vi "fpga_ARC Filter Info.vi"(1 "resample position [U64.16]":fxp<+,64,16>, 2 "stepsize [U64.8]":fxp<+,64,8>, 4 "input valid":bool, 6 "ARC Constants":T1={"bufsize"=512, "bufsize-1"=511, "NChan"=8, "NChan-1"=7, "1/2SymPeriods"=10, "Neg1/2SymPeriods"=-10, "polyOrder-1"=4, "maxDec-1"=24}, 7 "ready for output":bool) -> (13 "ready for input":bool, 14 "Initial position":u16, 15 "Initial offset":u32, 16 "Number of taps":u16, 17 "filterStepSize[U32.0]":u32 format="%08x", 18 "output valid":bool)   [LabVIEW 2011, in "NI_EP_Resample_FPGA.lvlib"]
uses:
  <vilib>/addons/Electrical Power/PQ/Resampling/NI_EP_Resample_FPGA.lvlib
  <vilib>/rvi/FXPMathLib/FxpConvert/subVIs/nifxpmath_Convert_SimConfig.ctl
  <vilib>/fxp/LVFixedPointQuantizationPolicyTypeDef.ctl
  <vilib>/fxp/LVFixedPointOverflowPolicyTypeDef.ctl
  <vilib>/rvi/FXPMathLib/FxpDiv/subVIs/nifxpmath_Div_SimConfig.ctl
  <vilib>/rvi/FXPMathLib/FxpConvert/simVIs/DllFxpConvertTemp_sub.vi
  <vilib>/rvi/FXPMathLib/FxpDiv/simVIs/DllFxpDivTemp_sub.vi
  <vilib>/rvi/FXPMathLib/FxpConvert/XNode/nifxpmath_Convert.xnode
  <vilib>/rvi/FXPMathLib/basic elements/FxpDiscreteDelay/XNode/nifxpmath_DiscreteDelay.xnode
  <vilib>/rvi/Arithmetic/AddSubMult/XNode/nirviSatArithmetic.xnode
  <vilib>/rvi/FXPMathLib/basic elements/FxpAddSub/XNode/nifxpmath_AddSub.xnode
  <vilib>/rvi/FXPMathLib/FxpReciprocal/XNode/nifxpmath_Reciprocal.xnode
  <vilib>/rvi/FXPMathLib/FxpDiv/XNode/nifxpmath_Div.xnode
  <vilib>/rvi/FXPMathLib/sim/FxpSim.dll
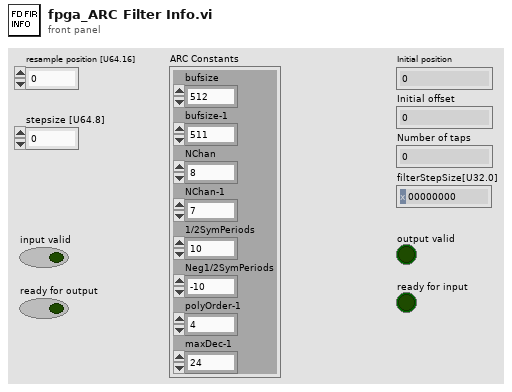
[diagram p1: front panel]
types:
  T1 = cluster{"bufsize":u16, "bufsize-1":u16, "NChan":u8, "NChan-1":u8, "1/2SymPeriods":i8, "Neg1/2SymPeriods":i8, "polyOrder-1":u8, "maxDec-1":u8}
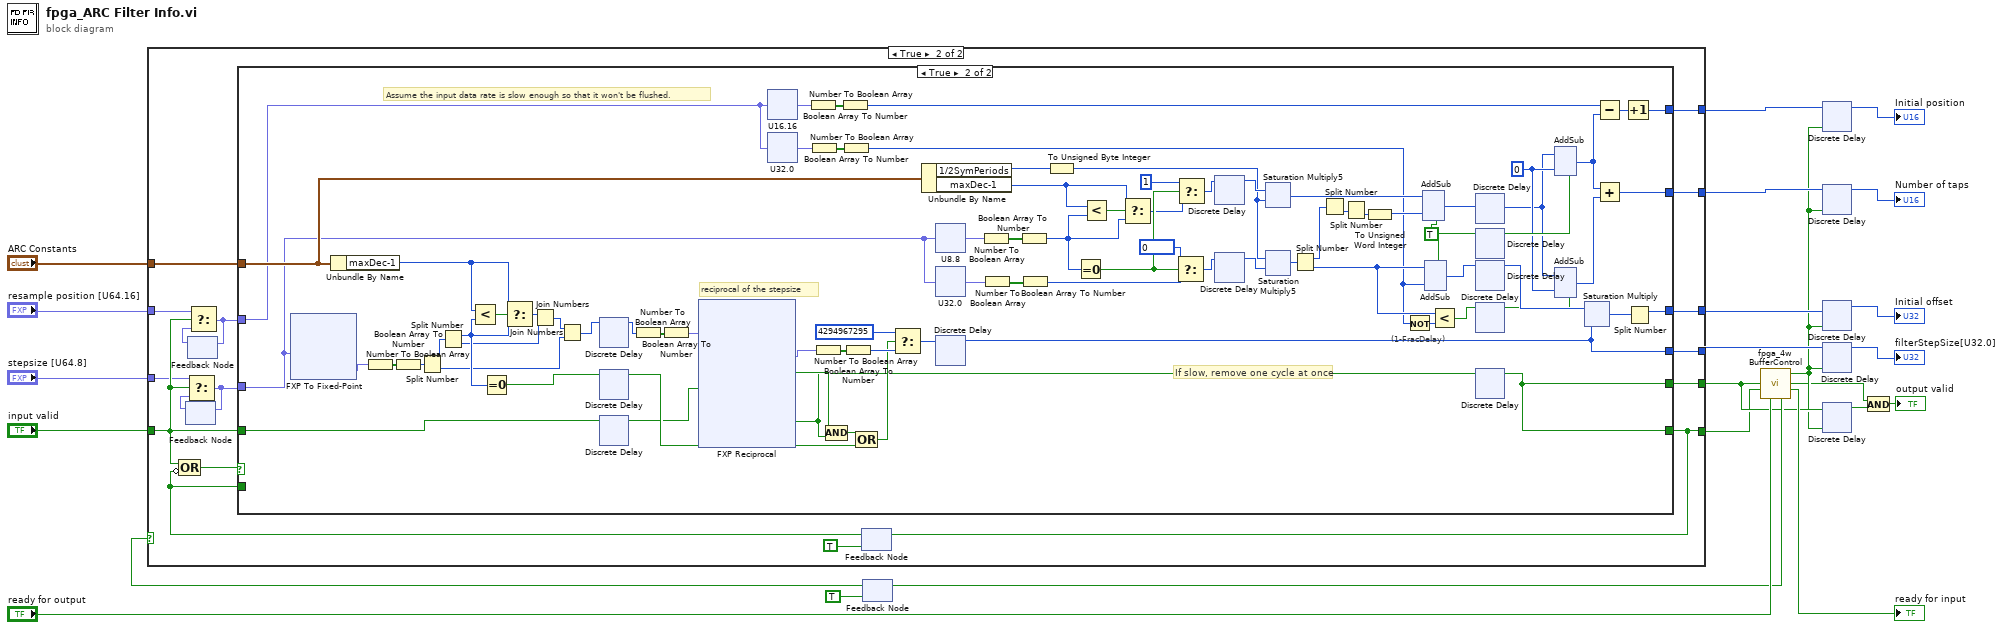
[diagram p0: block diagram]
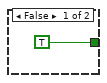
[diagram p3: hidden frame]
diagram:
  n1 = feedback #1(TRUE ("logic enable")) -> (w18:bool)
  n2 = case shown="True" w18 {
    tunnel: [_ w39] -> w8
    tunnel: "resample position [U64.16]" -> [_ w30]
    tunnel: "ARC Constants" -> [_ w40]
    tunnel: "input valid" -> [_ w26]
    tunnel: [_ w35] -> w7
    tunnel: [_ w31] -> w6
    tunnel: [_ w36] -> w11
    tunnel: [_ w37] -> w10
    tunnel: [_ w38] -> w9
    tunnel: "stepsize [U64.8]" -> [_ w25]
    frame False {
    }
    frame True {
      n3 = feedback #2() -> (w27:fxp<+,64,8>)  [unwired: 1 out]
      n4 = Select(t=w25, s=w26, f=w27) -> (s? t:f=w24:fxp<+,64,8>)
      n5 = feedback-in #2(w24) -> ()
      n6 = feedback #3() -> (w28:fxp<+,64,16>)  [unwired: 1 out]
      n7 = Select(t=w30, s=w26, f=w28) -> (s? t:f=w29:fxp<+,64,16>)
      n8 = feedback-in #3(w29) -> ()
      n9 = feedback #4(TRUE ("Q")) -> (w32:bool)
      n10 = Compound Arithmetic op=OR(w26, invert w32) -> (w33:bool)
      n11 = case shown="True" w33 {
        tunnel: [_ w46] -> w35
        tunnel: w40 -> [_ w58]
        tunnel: [_ w56] -> w39
        tunnel: [_ w55] -> w38
        tunnel: [_ w54] -> w37
        tunnel: [_ w51] -> w36
        tunnel: w32 -> [_ _]
        tunnel: [TRUE ("Q") w46] -> w31
        tunnel: w26 -> [_ w49]
        tunnel: w29 -> [_ w45]
        tunnel: w24 -> [_ w44]
        frame False {
        }
        frame True {
          w75 = u16 0 ("y")
          # "If slow, remove one cycle at once"
          # "(1-FracDelay)"
          # "Assume the input data rate is slow enough so that it won't be flushed."
          # "reciprocal of the stepsize"
          n12 = xnode "FXP To Fixed-Point"("x"=w44) -> ("y"=w120:fxp<+,32,8>)
          n13 = Unbundle By Name(w58) -> ("maxDec-1"=w110:u8)
          n14 = Number To Boolean Array(number=w120) -> (Boolean array=w119:bool[])
          n15 = Boolean Array To Number(Boolean array=w119) -> (number=w118:u32)
          n16 = Split Number(x=w118) -> (hi(x)=w117:u16, lo(x)=w111:u16)
          n17 = Split Number(x=w117) -> (hi(x)=w115:u8, lo(x)=w113:u8)
          n18 = Less?(x=w110, y=w115) -> (x < y?=w116:bool)
          n19 = Equal To 0?(x=w115) -> (x = 0?=w123:bool)
          n20 = Select(t=w110, s=w116, f=w115) -> (s? t:f=w114:u8)
          n21 = Join Numbers(hi=w114, lo=w113) -> ((hi.lo)=w112:u16)
          n22 = Join Numbers(hi=w112, lo=w111) -> ((hi.lo)=w122:u32)
          n23 = xnode "Discrete Delay"("D"=w122) -> ("Q"=w121:u32)
          n24 = xnode "Discrete Delay"("D"=w123) -> ("Q"=w103:bool)
          n25 = xnode "Discrete Delay"("D"=w49) -> ("Q"=w50:bool)
          n26 = Number To Boolean Array(number=w121) -> (Boolean array=w109:bool[])
          n27 = Boolean Array To Number(Boolean array=w109) -> (number=w108:fxp<+,32,8>)
          n28 = xnode "FXP Reciprocal"("x"=w108, "input valid"=w50) -> ("1/x"=w106:fxp<+,32,0>, "operation overflow"=w105:bool, "output valid"=w47:bool)  [unwired: 1 in, 1 out]
          n29 = xnode "U16.16"("x"=w45) -> ("y"=w62:fxp<+,16,16>)
          n30 = xnode "U32.0"("x"=w45) -> ("y"=w60:fxp<+,32,0>)
          n31 = Number To Boolean Array(number=w62) -> (Boolean array=w63:bool[])
          n32 = Number To Boolean Array(number=w60) -> (Boolean array=w61:bool[])
          n33 = Number To Boolean Array(number=w106) -> (Boolean array=w107:bool[])
          n34 = Compound Arithmetic op=AND(w105, w47) -> (w104:bool)
          n35 = Boolean Array To Number(Boolean array=w63) -> (number=w53:u16)
          n36 = Boolean Array To Number(Boolean array=w61) -> (number=w59:u32)
          n37 = Boolean Array To Number(Boolean array=w107) -> (number=w101:u32)
          n38 = Compound Arithmetic op=OR(w104, w103) -> (w99:bool)
          n39 = Select(t=u32 4294967295, s=w99, f=w101) -> (s? t:f=w102:u32)
          n40 = Unbundle By Name(w58) -> ("1/2SymPeriods"=w95:i8, "maxDec-1"=w42:u8)
          n41 = xnode "U8.8"("x"=w44) -> ("y"=w67:fxp<+,8,8>)
          n42 = xnode "U32.0"("x"=w44) -> ("y"=w65:fxp<+,32,0>)
          n43 = xnode "Discrete Delay"("D"=w102) -> ("Q"=w56:u32)
          n44 = Number To Boolean Array(number=w67) -> (Boolean array=w68:bool[])
          n45 = Number To Boolean Array(number=w65) -> (Boolean array=w66:bool[])
          n46 = Boolean Array To Number(Boolean array=w68) -> (number=w43:u8)
          n47 = Boolean Array To Number(Boolean array=w66) -> (number=w64:u32)
          n48 = To Unsigned Byte Integer(number=w95) -> (unsigned 8bit integer=w89:u8)
          n49 = Equal To 0?(x=w43) -> (x = 0?=w71:bool)
          n50 = Less?(x=w42, y=w43) -> (x < y?=w48:bool)
          n51 = Select(t=w42, s=w48, f=w43) -> (s? t:f=w70:u8)
          n52 = Select(t=u32 0, s=w71, f=w64) -> (s? t:f=w93:u32)
          n53 = Select(t=u8 1, s=w71, f=w70) -> (s? t:f=w90:u8)
          n54 = xnode "Discrete Delay"("D"=w90) -> ("Q"=w94:u8)
          n55 = xnode "Discrete Delay"("D"=w93) -> ("Q"=w88:u32)
          n56 = xnode ("Saturation Multiply5")("x"=w94, "y"=w89) -> ("x*y"=w83:u16)
          n57 = xnode ("Saturation Multiply5")("x"=w89, "y"=w88) -> ("x*y"=w87:u64)
          n58 = Split Number(x=w87) -> (hi(x)=w86:u32, lo(x)=w78:u32)
          n59 = Split Number(x=w86) -> (lo(x)=w85:u16)  [unwired: 1 out]
          n60 = Split Number(x=w85) -> (lo(x)=w84:u8)  [unwired: 1 out]
          n61 = To Unsigned Word Integer(number=w84) -> (unsigned 16bit integer=w82:u16)
          n62 = Not(x=w59) -> (.not. x?=w96:u32)
          n63 = xnode "AddSub"("x"=w83, "y"=w82, "carry-in"=TRUE ("Cin/Bin_n")) -> ("s"=w80:u16)  [unwired: 1 out]
          n64 = xnode "AddSub"("x"=w78, "y"=w59) -> ("s"=w77:u32, "borrow-out"=w79:bool)
          n65 = Less?(x=w78, y=w96) -> (x < y?=w98:bool)
          n66 = xnode "Discrete Delay"("D"=w80) -> ("Q"=w73:u16)
          n67 = xnode "Discrete Delay"("D"=w79) -> ("Q"=w76:bool)
          n68 = xnode "Discrete Delay"("D"=w77) -> ("Q"=w92:u32)
          n69 = xnode "Discrete Delay"("D"=w98) -> ("Q"=w72:bool)
          n70 = xnode "Discrete Delay"("D"=w47) -> ("Q"=w46:bool)
          n71 = xnode "AddSub"("x"=w73, "y"=w75, "borrow-in"=w76) -> ("s"=w57:u16)  [unwired: 1 out]
          n72 = xnode "AddSub"("x"=w73, "y"=w75, "borrow-in"=w72) -> ("s"=w74:u16)  [unwired: 1 out]
          n73 = xnode ("Saturation Multiply")("x"=w92, "y"=w56) -> ("x*y"=w91:u64)
          n74 = Subtract(x=w53, y=w57) -> (x-y=w52:u16)
          n75 = Add(x=w57, y=w74) -> (x+y=w54:u16)
          n76 = Increment(x=w52) -> (x+1=w51:u16)
          n77 = Split Number(x=w91) -> (hi(x)=w55:u32)  [unwired: 1 out]
        }
      }
      n78 = feedback-in #4(w31) -> ()
    }
  }
  n79 = call <vilib>:"fpga_4w BufferControl.vi"("DR"=w7, "RFI"=w6, "RFO"="ready for output") -> ("buff enable"=w5:bool, "output valid"=w2:bool, "ready for input"=→"ready for input":bool, "logic enable"=w19:bool)  [unwired: 9 in]
  n80 = feedback-in #1(w19) -> ()
  n81 = xnode "Discrete Delay"("D"=w11, "enable"=w5) -> ("Q"=→"Initial position":u16)
  n82 = xnode "Discrete Delay"("D"=w10, "enable"=w5) -> ("Q"=→"Number of taps":u16)
  n83 = xnode "Discrete Delay"("D"=w9, "enable"=w5) -> ("Q"=→"Initial offset":u32)
  n84 = xnode "Discrete Delay"("D"=w8, "enable"=w5) -> ("Q"=→"filterStepSize[U32.0]":u32)
  n85 = xnode "Discrete Delay"("D"=w7, "enable"=w5) -> ("Q"=w12:bool)
  n86 = Compound Arithmetic op=AND(w2, w12) -> (→"output valid":bool)
